vi "Operation UI.vi"(0 "A":dbl, 5 "B":dbl, 7 "Calculate":bool, 9 "DVR In":refnum<data-value>, 11 "Error In":errorcluster) -> (4 "C":dbl, 10 "DVR  Out":refnum<data-value>, 15 "Error Out":errorcluster)   [LabVIEW 2023, in "Subtract.lvclass"]
doc: "The VI contains the addition operation UI that accepts two input numbers and performs subtraction operation and displays the output when user clicks calculate button"
uses:
  Subtract.lvclass
  Arithemtic Operation/Arithemetic Operation.lvclass
  Typedef/User Event Operations.ctl
panel:
  # "SUBTRACTION"
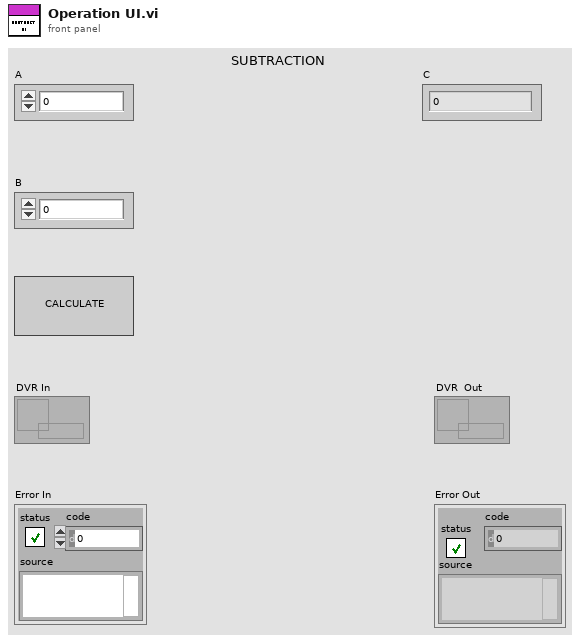
[diagram p1: front panel]
types:
  T1 = typedef "User Event Operations.ctl" = enum16{"Obtain", "Generate", "Destroy"}
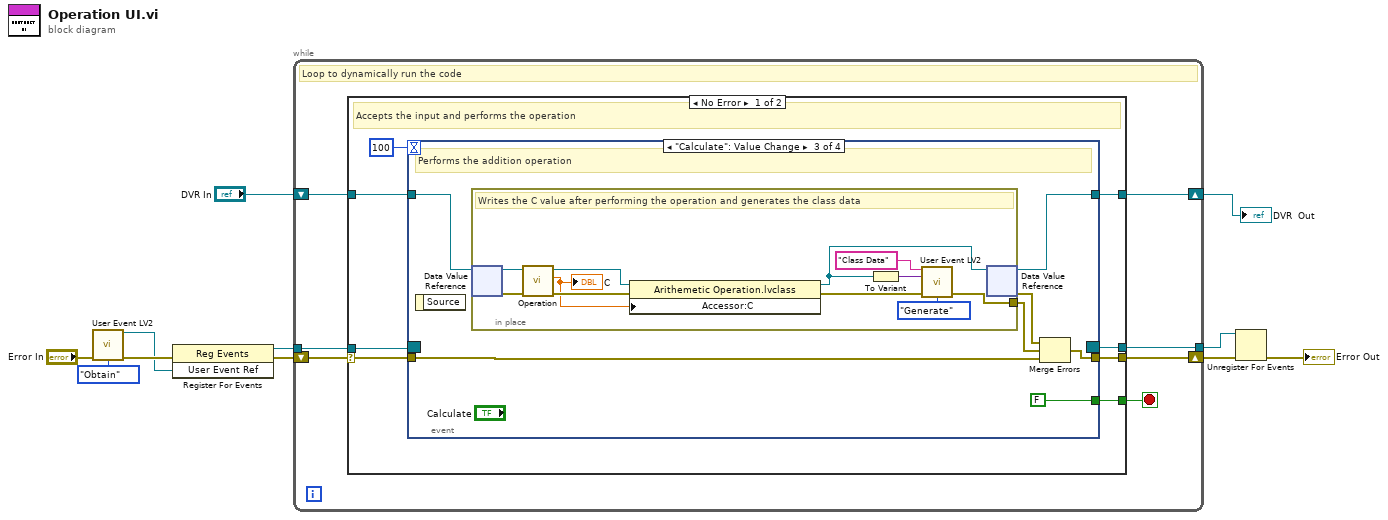
[diagram p0: block diagram]
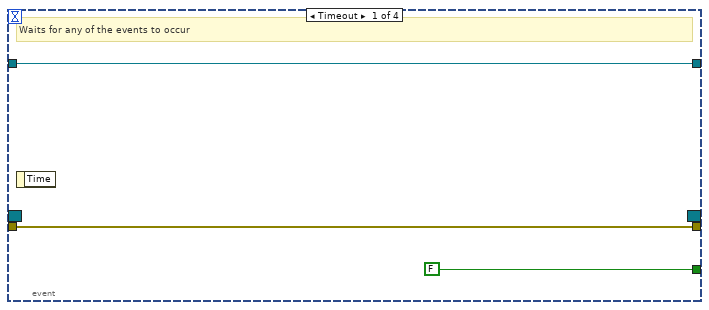
[diagram p2: hidden frame]
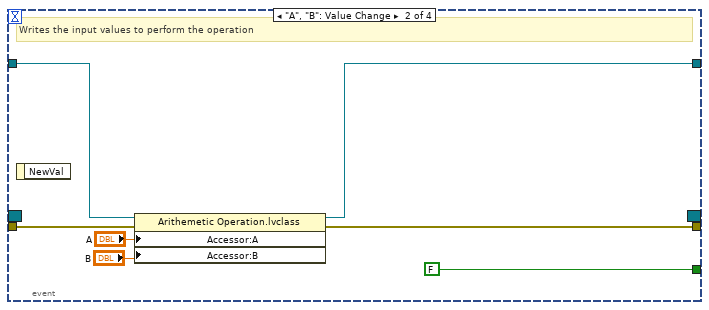
[diagram p3: hidden frame]
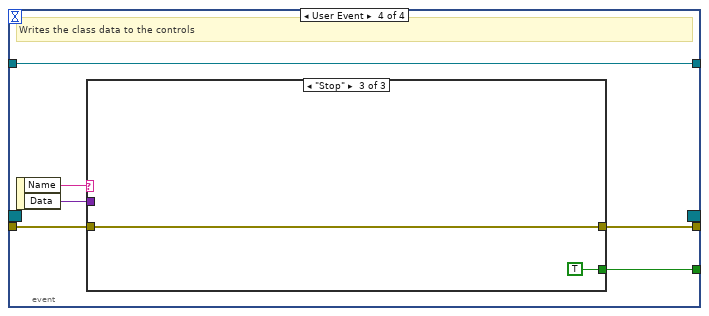
[diagram p4: hidden frame]
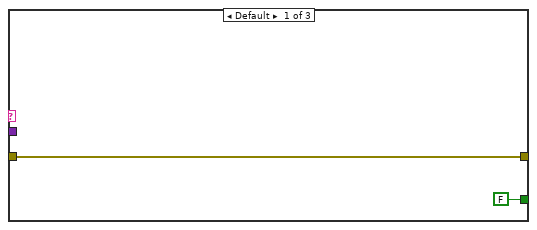
[diagram p5: hidden frame]
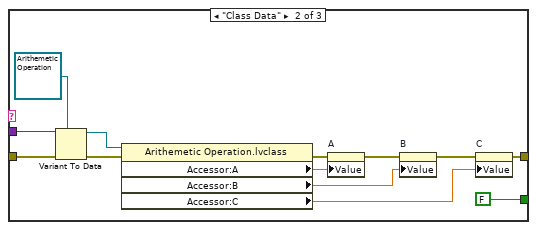
[diagram p6: hidden frame]
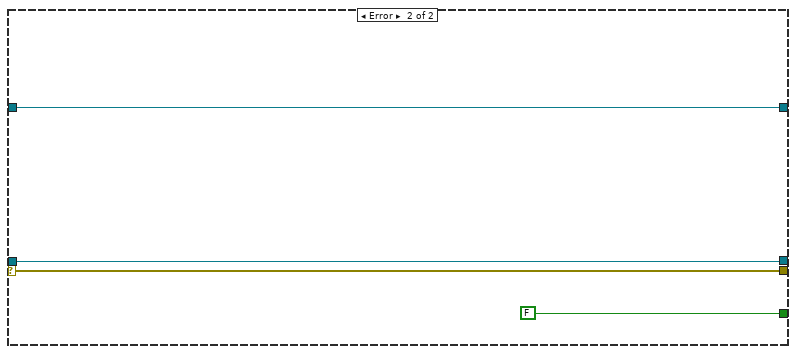
[diagram p7: hidden frame]
diagram:
  n1 = call "User Event LV2.vi"("Error In"="Error In", "Operation"=User_Event_Operations."Obtain") -> ("User Event Ref"=w2:refnum<user-event>, "Error Out"=w3:errorcluster)  [unwired: 12 in]
  n2 = register-events(error in=w3, w2) -> (reference out=w8:refnum<event-registration>, error out=w9:errorcluster)  [unwired: 1 in]
  n3 = while {
    shift-right: [w17] -> w11
    shift-left: w9 -> [w18]
    shift-right: [w15] -> w5
    shift-left: "DVR In" -> [w16]
    tunnel: w8 -> [w14]
    tunnel: [w13] -> w6
    stop <- w12 stop-if-true
    # "Loop to dynamically run the code"
    n4 = case shown="No Error" w18 {
      selector: w18 -> [w24 w81]
      tunnel: [w23 w81] -> w17
      tunnel: [w25 w80] -> w15
      tunnel: w16 -> [w26 w80]
      tunnel: w14 -> [w21 w79]
      tunnel: [w20 w79] -> w13
      tunnel: [w19 FALSE] -> w12
      frame No Error {
        # "Accepts the input and performs the operation"
        n5 = event shown="[2] \"Calculate\": Value Change" {
          selector: w21 -> [_ _ _ _]
          dyn-events: [_ _ _ _] -> w20
          timeout: 100 -> [_ _ _ _]
          tunnel: [w29 w31 w41 w60] -> w25
          tunnel: w26 -> [w29 w34 w42 w60]
          tunnel: w24 -> [w28 w36 w40 w59]
          tunnel: [w28 w35 w37 w58] -> w23
          tunnel: [FALSE FALSE FALSE w57] -> w19
          event Timeout {
            # "Waits for any of the events to occur"
            n6 = event-data() -> ()  [unwired: 1 in, 1 out]
          }
          event "A", "B": Value Change {
            # "Writes the input values to perform the operation"
            n7 = event-data() -> ()  [unwired: 1 in, 1 out]
            n8 = property class="Arithemetic Operation.lvclass"(reference=w34, error in=w36, "Accessor:A"="A", "Accessor:B"="B") -> (reference out=w31:refnum<data-value>, error out=w35:errorcluster)
          }
          event "Calculate": Value Change {
            # "Performs the addition operation"
            n9 = event-data() -> ()  [unwired: 1 in, 1 out]
            n10 = in-place {
              in-place-border: [w45] -> w39
              # "Writes the C value after performing the operation and generates the class data"
              n11 = in-place-dvr #1(w42) -> (w51:refnum<class "Arithemetic Operation.lvclass">, w50:errorcluster)
              n12 = call-dynamic "Operation.vi"("Error In"=w50, "Arithemetic Operation in"=w51) -> ("Error Out"=w54:errorcluster, "C"=w52:dbl, "Arithemetic Operation out"=w53:refnum<class "Arithemetic Operation.lvclass">)  [unwired: 7 in]
              "C" <- w52
              n13 = property class="Arithemetic Operation.lvclass"(reference=w53, error in=w54, "Accessor:C"=w52) -> (reference out=w44:refnum<class "Arithemetic Operation.lvclass">, error out=w46:errorcluster)
              n14 = To Variant(anything=w44) -> (Variant=w49:variant)
              n15 = call "User Event LV2.vi"("Event Name"="Class Data", "Data"=w49, "Error In"=w46, "Operation"=User_Event_Operations."Generate") -> ("Error Out"=w45:errorcluster)  [unwired: 10 in, 1 out]
              n16 = in-place-dvr #1(w44) -> (w41:refnum<data-value>, w38:errorcluster)
            }
            n17 = Merge Errors(w38, w39, w40) -> (w37:errorcluster)
          }
          event User Event {
            # "Writes the class data to the controls"
            n18 = event-data() -> ("Name"=w56:string, "Data"=w55:variant)  [unwired: 1 in]
            n19 = case shown="\"Stop\"" w56 {
              tunnel: w59 -> [w62 w75 w77]
              tunnel: [w62 w71 w77] -> w58
              tunnel: [FALSE FALSE TRUE] -> w57
              tunnel: w55 -> [_ w65 _]
              frame Default {
              }
              frame "Class Data" {
                n20 = Variant To Data(error in=w75, type=refnum<class "Arithemetic Operation.lvclass"> refnum ("reference out"), Variant=w65) -> (data=w64:refnum<class "Arithemetic Operation.lvclass">, error out=w66:errorcluster)
                n21 = property class="Arithemetic Operation.lvclass"(reference=w64, error in=w66) -> (error out=w74:errorcluster, "Accessor:A"=w70:dbl, "Accessor:B"=w69:dbl, "Accessor:C"=w68:dbl)  [unwired: 1 out]
                n22 = property on="A" class="DigNum (strict)"(error in=w74, "Value"=w70) -> (error out=w73:errorcluster)  [unwired: 1 in, 1 out]
                n23 = property on="B" class="DigNum (strict)"(error in=w73, "Value"=w69) -> (error out=w72:errorcluster)  [unwired: 1 in, 1 out]
                n24 = property on="C" class="DigNum (strict)"(error in=w72, "Value"=w68) -> (error out=w71:errorcluster)  [unwired: 1 in, 1 out]
              }
              frame "Stop" {
              }
            }
          }
        }
      }
      frame Error {
      }
    }
  }
  "DVR  Out" <- w5
  n25 = Unregister For Events(event registration refnum=w6, error in=w11) -> (error out=→"Error Out":errorcluster)
